vi "TD_Open_Connection.vi"(8 "Error In":errorcluster, 11 "Access Key":string) -> (0 "Error Out":errorcluster, 3 "TekDrive Session":T1)   [LabVIEW 2018]
uses:
  Controls/TekDriveSession.ctl
  <vilib>/httpClient/ClientHandle.ctl
  <vilib>/httpClient/LabVIEWHTTPClient.lvlib
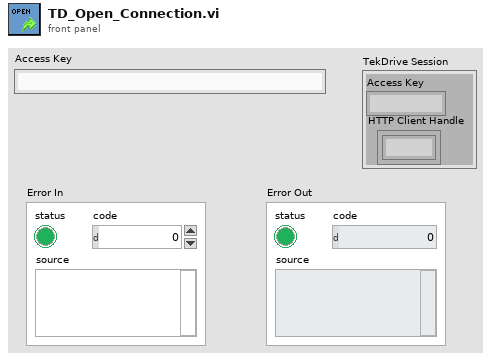
[diagram p1: front panel]
types:
  T1 = typedef "TekDriveSession.ctl" = cluster{"Access Key":string, "HTTP Client Handle":T2}
  T2 = typedef "LabVIEWHTTPClient.lvlib/ClientHandle.ctl" = refnum<k1>
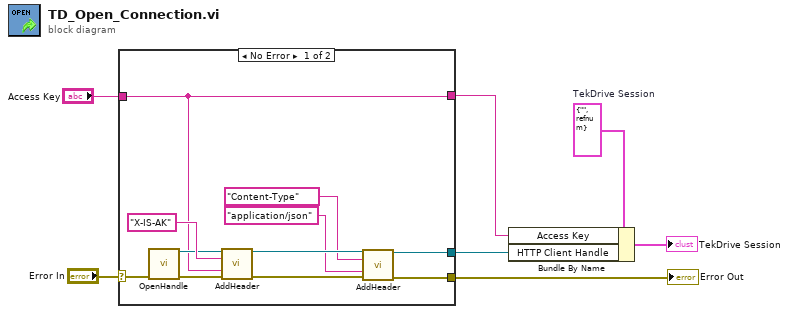
[diagram p0: block diagram]
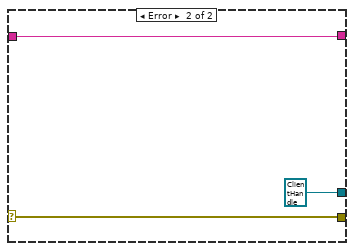
[diagram p2: hidden frame]
diagram:
  w4 = T1 {"Access Key"="", "HTTP Client Handle"=refnum}  # TekDrive Session
  n1 = case shown="No Error" "Error In" {
    selector: "Error In" -> [w18 w21]
    tunnel: "Access Key" -> [w8 w19]
    tunnel: [w10 T2 refnum ("client handle out")] -> w2
    tunnel: [w9 w21] -> w5
    tunnel: [w8 w19] -> w3
    frame No Error {
      n2 = call <vilib>:"OpenHandle.vi"("error in (no error)"=w18) -> ("client handle out"=w15:T2, "error out"=w17:errorcluster)  [unwired: 13 in]
      n3 = call <vilib>:"AddHeader.vi"("client handle"=w15, "header"="X-IS-AK" ("Access Key"), "value"=w8, "error in (no error)"=w17) -> ("client handle out"=w14:T2, "error out"=w13:errorcluster)  [unwired: 10 in]
      n4 = call <vilib>:"AddHeader.vi"("client handle"=w14, "header"="Content-Type", "value"="application/json", "error in (no error)"=w13) -> ("client handle out"=w10:T2, "error out"=w9:errorcluster)  [unwired: 10 in]
    }
    frame Error {
    }
  }
  "Error Out" <- w5
  n5 = Bundle By Name(cluster=w4, "Access Key"=w3, "HTTP Client Handle"=w2) -> (→"TekDrive Session":T1)
